vi "CMFB restarts (FPGA).vi"() -> ()   [LabVIEW 2019]
uses:
  <vilib>/rvi/Emulation/niFpgaGetClockAttributes.vi
  <vilib>/rvi/Emulation/niFpgaSctlEmulationGetInTimedLoop.vi
  <vilib>/rvi/Emulation/niFpgaEmulationReportErrorSimple.vi
  <vilib>/rvi/Emulation/niFpgaProcessEmulError.vi
  <vilib>/rvi/Emulation/niFpgaCriticalErrorInLSC.vi
panel:
  in  "Pump Starts Enable":bool
  in  "Reset Pump Starts":bool
  out "Pump On States":bool[](array[boolean])
  out "Timers (ms)":u32[](array[numeric])
  out "Pump Starts":u32[](array[numeric])
  in  "Off Current Thresh":fxp<+/-,28,17>
  in  "Min Off Time":u32
  in  "Min On Time":u32
  in  "On Current Thresh":fxp<+/-,28,17>
  in  "Controller Currents":fxp<+/-,28,17>[](array[numeric])=[0.0, 0.0, 0.0, 0.0, 0.0, 0.0]
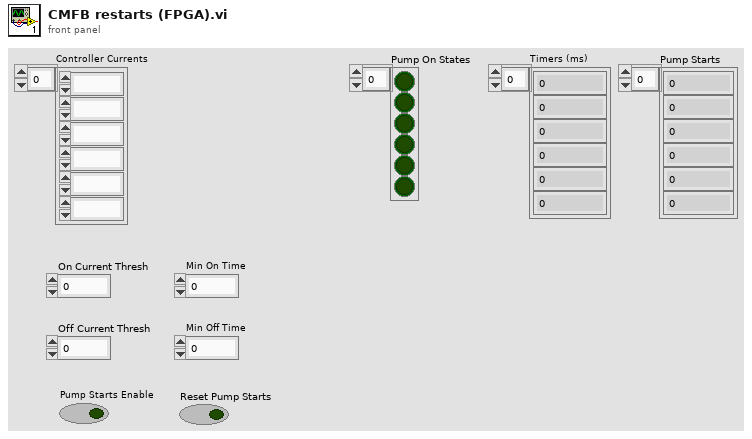
[diagram p1: front panel]
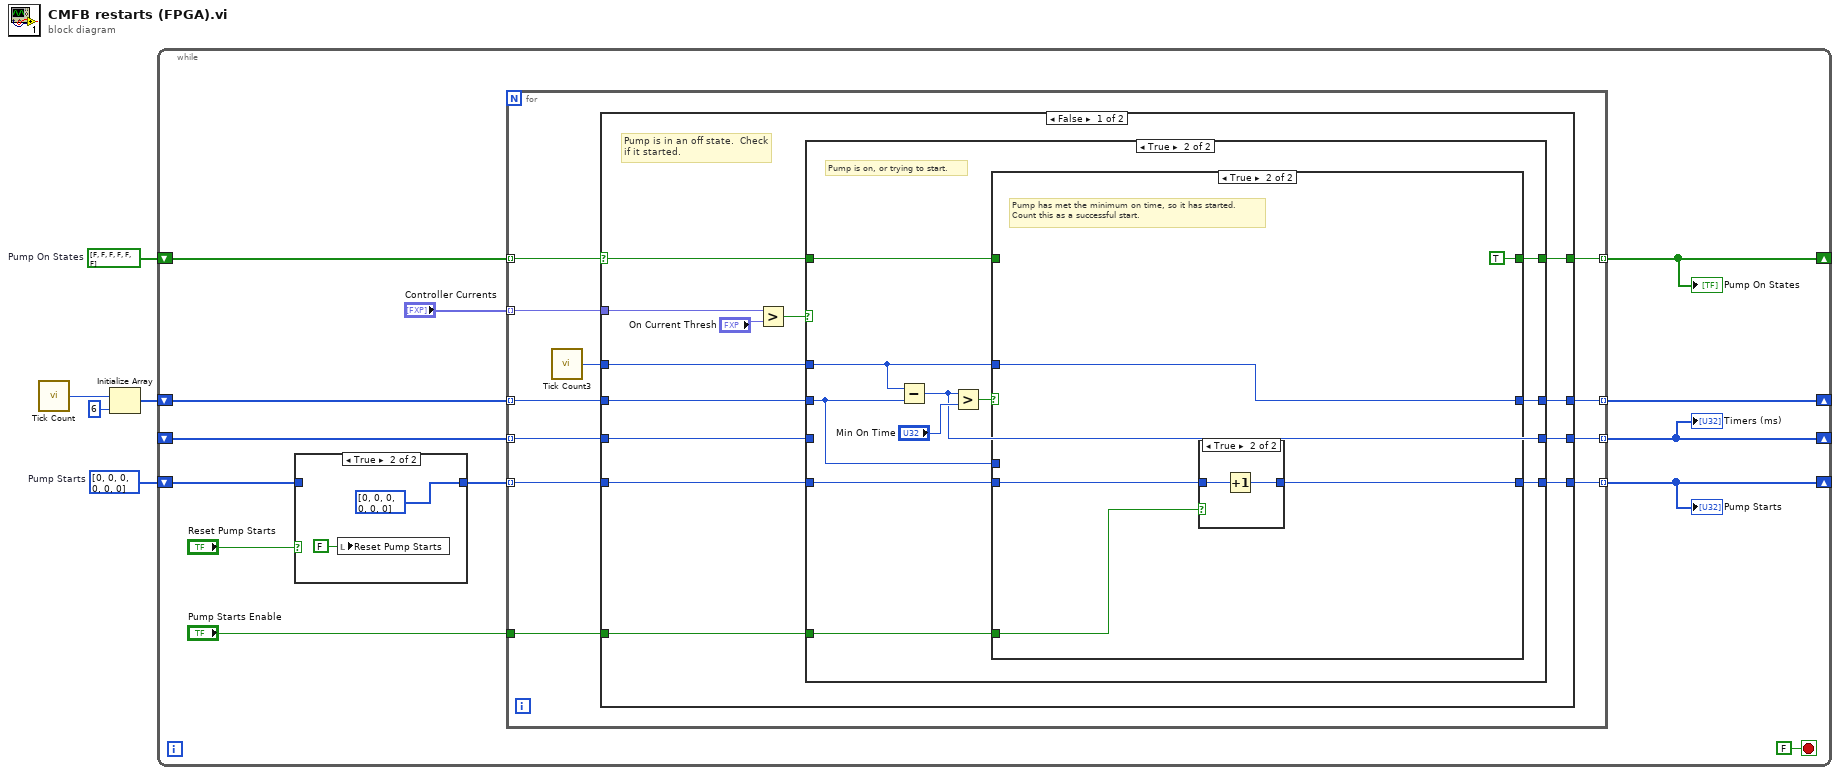
[diagram p0: block diagram]
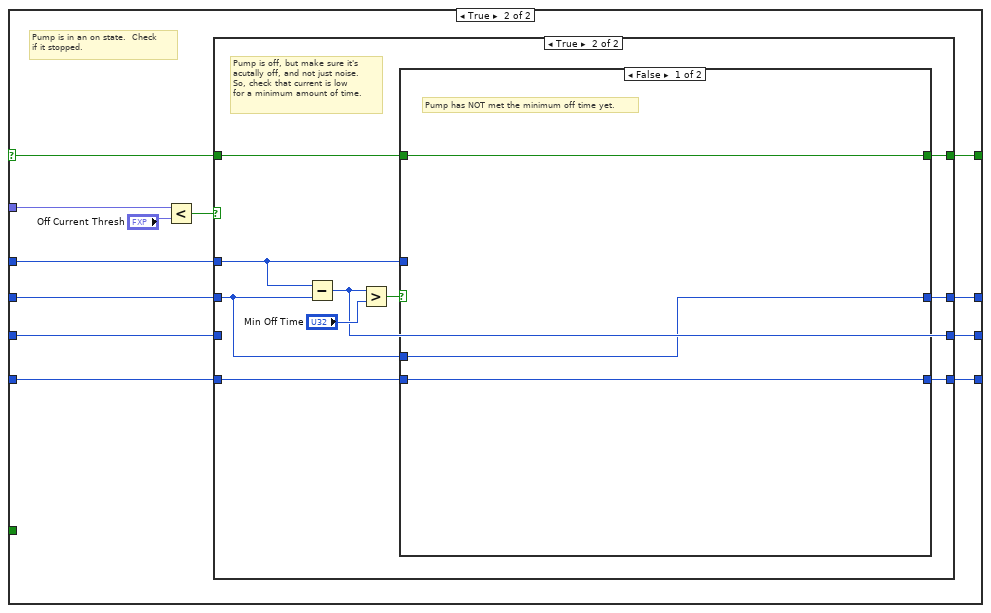
[diagram p6: hidden frame]
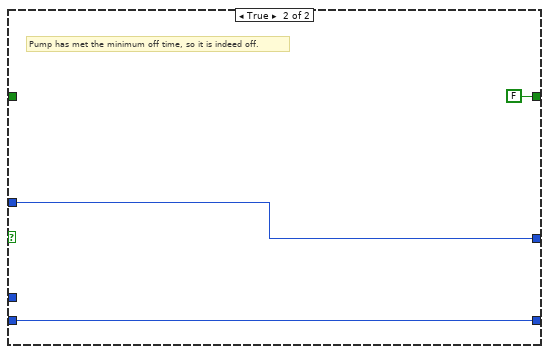
[diagram p8: hidden frame]
diagram:
  w1 = bool[] [FALSE, FALSE, FALSE, FALSE, FALSE, FALSE]  # Pump On States
  w2 = u32[] [0, 0, 0, 0, 0, 0]  # Pump Starts
  n1 = call "Tick Count"() -> ("Tick Count(mSec)"=w5:u32)
  n2 = Initialize Array(w5, 6 ("dimension size")) -> (w3:u32[])
  n3 = while {
    shift-right: [w13] -> _
    shift-left: w3 -> [w17]
    shift-right: [w16] -> _
    shift-left: w2 -> [w9]
    shift-right: [w14] -> _
    shift-left: w1 -> [w15]
    shift-right: [w12] -> _
    shift-left: _ -> [w11]
    stop <- FALSE stop-if-true
    n4 = case shown="True" "Reset Pump Starts" {
      tunnel: w9 -> [w19 _]
      tunnel: [w19 u32[] [0, 0, 0, 0, 0, 0] ("Pump Starts")] -> w7
      frame False {
      }
      frame True {
        n5 = local write "Reset Pump Starts"(FALSE ("Reset Pump Starts")) -> ()
      }
    }
    n6 = for {
      tunnel: "Controller Currents" -> [w32] mode=indexing
      tunnel: w17 -> [w31] mode=indexing
      tunnel: w7 -> [w30] mode=indexing
      tunnel: [w29] -> w16 mode=indexing
      tunnel: w15 -> [w27] mode=indexing
      tunnel: [w28] -> w14 mode=indexing
      tunnel: [w25] -> w13 mode=indexing
      tunnel: [w24] -> w12 mode=indexing
      tunnel: w11 -> [w23] mode=indexing
      tunnel: "Pump Starts Enable" -> [w22]
      n7 = call "Tick Count3"() -> ("Tick Count(mSec)"=w26:u32)
      n8 = case shown="False" w27 {
        selector: w27 -> [w38 w76]
        tunnel: w32 -> [w45 w83]
        tunnel: w31 -> [w43 w81]
        tunnel: w30 -> [w41 w79]
        tunnel: [w40 w78] -> w29
        tunnel: [w39 w77] -> w28
        tunnel: w26 -> [w37 w75]
        tunnel: [w36 w74] -> w25
        tunnel: [w35 w73] -> w24
        tunnel: w23 -> [w34 w72]
        tunnel: w22 -> [w33 _]
        frame False {
          # "Pump is in an off state.  Check\nif it started."
          n9 = Greater?(x=w45, y="On Current Thresh") -> (0:w42:bool)
          n10 = case shown="True" w42 {
            tunnel: w43 -> [_ w52]
            tunnel: w41 -> [w47 w58]
            tunnel: [w47 w57] -> w40
            tunnel: w38 -> [w49 w56]
            tunnel: [w49 w55] -> w39
            tunnel: w37 -> [w48 w53]
            tunnel: [w48 w54] -> w36
            tunnel: [w46 w51] -> w35
            tunnel: w34 -> [w46 _]
            tunnel: w33 -> [_ w50]
            frame False {
              # "Pump is off."
            }
            frame True {
              # "Pump is on, or trying to start."
              n11 = Subtract(x=w53, y=w52) -> (x-y=w51:u32)
              n12 = Greater?(x=w51, y="Min On Time") -> (0:w59:bool)
              n13 = case shown="True" w59 {
                tunnel: w58 -> [w63 w68]
                tunnel: [w63 w67] -> w57
                tunnel: w56 -> [w61 _]
                tunnel: [w61 TRUE] -> w55
                tunnel: [w62 w65] -> w54
                tunnel: w53 -> [_ w65]
                tunnel: w52 -> [w62 _]
                tunnel: w50 -> [_ w64]
                frame False {
                  # "Pump has NOT met the minimum on time yet."
                }
                frame True {
                  # "Pump has met the minimum on time, so it has started.\nCount this as a successful start."
                  n14 = case shown="True" w64 {
                    tunnel: w68 -> [w69 w71]
                    tunnel: [w69 w70] -> w67
                    frame False {
                    }
                    frame True {
                      n15 = Increment(x=w71) -> (x+1=w70:u32)
                    }
                  }
                }
              }
            }
          }
        }
        frame True {
          # "Pump is in an on state.  Check\nif it stopped."
          n16 = Less?(x=w83, y="Off Current Thresh") -> (x < y?=w80:bool)
          n17 = case shown="True" w80 {
            tunnel: w81 -> [_ w89]
            tunnel: w79 -> [w86 w95]
            tunnel: [w86 w94] -> w78
            tunnel: w76 -> [w85 w93]
            tunnel: [w85 w92] -> w77
            tunnel: w75 -> [w87 w90]
            tunnel: [w87 w91] -> w74
            tunnel: [w84 w88] -> w73
            tunnel: w72 -> [w84 _]
            frame False {
              # "Pump is in on."
            }
            frame True {
              # "Pump is off, but make sure it's\nacutally off, and not just noise.\nSo, check that current is low\nfor a minimum amount of time."
              n18 = Subtract(x=w90, y=w89) -> (x-y=w88:u32)
              n19 = Greater?(x=w88, y="Min Off Time") -> (0:w96:bool)
              n20 = case shown="False" w96 {
                tunnel: w95 -> [w99 w102]
                tunnel: [w99 w102] -> w94
                tunnel: w93 -> [w100 _]
                tunnel: [w100 FALSE] -> w92
                tunnel: [w98 w101] -> w91
                tunnel: w90 -> [_ w101]
                tunnel: w89 -> [w98 _]
                frame False {
                  # "Pump has NOT met the minimum off time yet."
                }
                frame True {
                  # "Pump has met the minimum off time, so it is indeed off."
                }
              }
            }
          }
        }
      }
    }
    "Pump Starts" <- w16
    "Timers (ms)" <- w12
    "Pump On States" <- w14
  }
